vi "Test_Ampere_Meting.vi"() -> ()   [LabVIEW 2016]
panel:
  in  "stop":bool
  out "Waveform Chart":dynamicdata(graph)
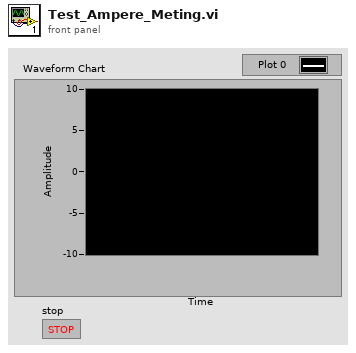
[diagram p1: front panel]
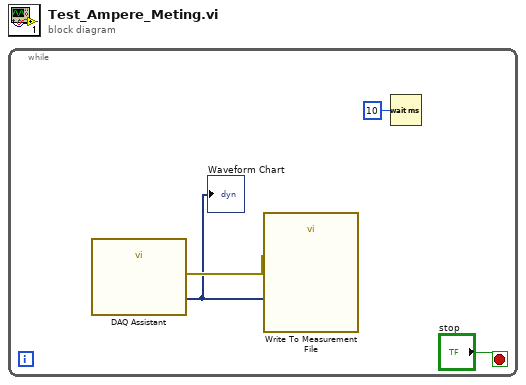
[diagram p0: block diagram]
diagram:
  n1 = while {
    stop <- "stop" stop-if-true
    n2 = call "DAQ Assistant"() -> ("data"=w2:dynamicdata, "error out"=w4:errorcluster)  [unwired: 17 in, 1 out]
    "Waveform Chart" <- w2
    n3 = call "Write To Measurement File"("Signals"=w2, "error in (no error)"=w4) -> ()  [unwired: 15 in, 3 out]
    n4 = Wait (ms)(milliseconds to wait=u32 10) -> ()  [unwired: 1 out]
  }
